vi "Perform Action.vi"(8 "error in":errorcluster, 10 "Input":variant, 11 "IPerform Action in":refnum<class "IPerform Action.lvclass">) -> (0 "error out":errorcluster, 2 "Output":variant, 3 "IPerform Action out":refnum<class "IPerform Action.lvclass">)   [LabVIEW 2023, in "IPerform Action.lvclass"]
uses:
  IPerform Action.lvclass
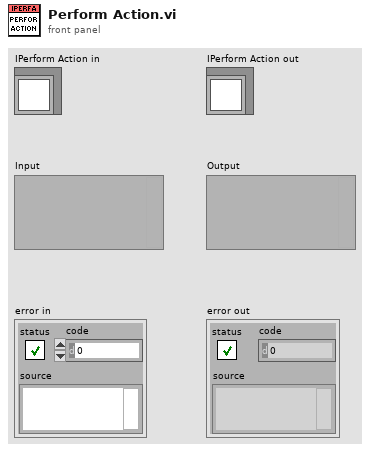
[diagram p1: front panel]
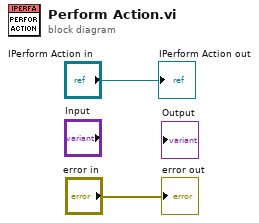
[diagram p0: block diagram]
diagram:
  "error out" <- "error in"
  "IPerform Action out" <- "IPerform Action in"
